vi "IAmGLF-NotARefnum.vi"(11 "Window in":refnum<class "Window.lvclass">) -> (2 "Not A Valid Refnum?":bool=TRUE, 3 "Window out":refnum<class "Window.lvclass">)   [LabVIEW 2020, in "GLF.lvlib" / "Window.lvclass"]
doc: "<B>Summary</B>\nReturns <B>True</B> if the class is invalid."
uses:
  Window.lvclass
  Window.lvclass/Window.ctl
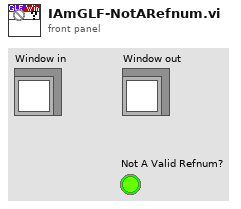
[diagram p1: front panel]
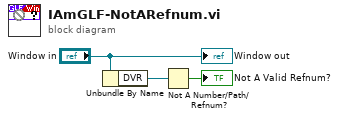
[diagram p0: block diagram]
diagram:
  n1 = Unbundle By Name("Window in") -> ("DVR"=w2:refnum<data-value>)
  n2 = Not A Number/Path/Refnum?(number/path/refnum=w2) -> (NaN/Path/Refnum?=→"Not A Valid Refnum?":bool)
  "Window out" <- "Window in"
